vi "GlobalVI.vi"() -> ()   [LabVIEW 2016]
panel:
  in  "position":cluster{"x":dbl, "y":dbl, "z":dbl}
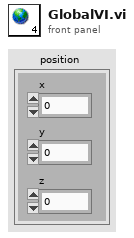
[diagram p1: front panel]
diagram:
